vi "Verify Quotes.vi"(10 "String In":string) -> (2 "Quote Verified String Out":string)   [LabVIEW 2016, in "QPA Measurement.lvlib" / "QPA Measurement.lvclass"]
uses:
  QPA Measurement.lvclass
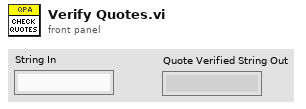
[diagram p1: front panel]
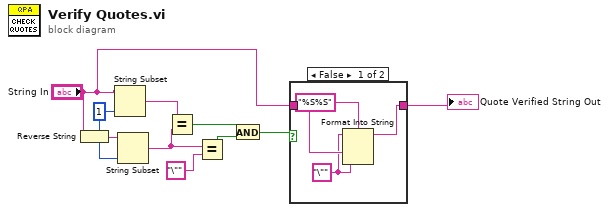
[diagram p0: block diagram]
diagram:
  w2 = 1 ("length (rest)")
  n1 = Reverse String(1:"String In") -> (0:w10:string)
  n2 = String Subset(string="String In", length (rest)=w2) -> (substring=w9:string)  [unwired: 1 in]
  n3 = String Subset(string=w10, length (rest)=w2) -> (substring=w8:string)  [unwired: 1 in]
  n4 = Equal?(x=w9, y=w8) -> (x = y?=w5:bool)
  n5 = Equal?(x=w8, y="\"") -> (x = y?=w6:bool)
  n6 = And(x=w5, y=w6) -> (x .and. y?=w4:bool)
  n7 = case shown="False" w4 {
    tunnel: [w12 w15] -> w1
    tunnel: "String In" -> [w14 w15]
    frame False {
      w13 = "\"" ("String In")
      n8 = Format Into String(format string="%S%S", initial string=w13, w14, w13) -> (resulting string=w12:string)  [unwired: 1 in, 1 out]
    }
    frame True {
    }
  }
  "Quote Verified String Out" <- w1
